vi "OpenBling.vi"(4 "OfflineMode":bool, 6 "Synchronous":bool=TRUE, 7 "Value Width":enum16{"4-bit", "8-bit"}(ring), 8 "error in (no error)":errorcluster, 9 "Chain Setup":cluster{"ChainNumber":u8, "numLeds":u8}[](array[cluster]), 10 "Reset on open?":bool, 11 "Serial Port":refnum<visa-resource-name>) -> (0 "error out":errorcluster, 3 "ControlState":T1 {"ChainMask" format="0x%02x"})   [LabVIEW 2023, in "ArduinoSerialBling.lvlib"]
uses:
  ArduinoSerialBling.lvlib
  ControlState.ctl
  ChainState.ctl
  <vilib>/Instr/_visa.llb/VISA Flush IO Buffer Mask.ctl
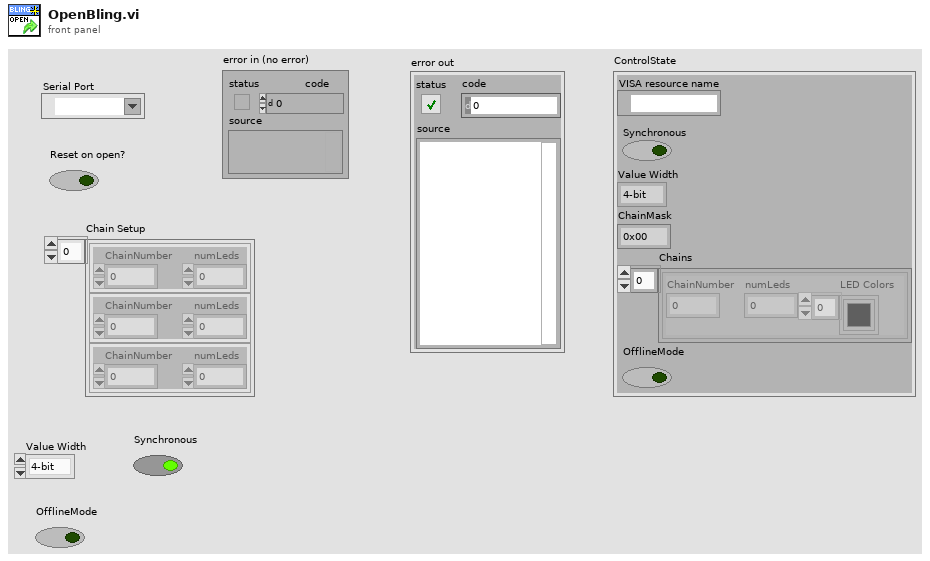
[diagram p1: front panel]
types:
  T1 = typedef "ArduinoSerialBling.lvlib/ControlState.ctl" = cluster{"VISA resource name":refnum<visa-resource-name>, "Synchronous":bool, "Value Width":enum16{"4-bit", "8-bit"}, "ChainMask":u8, "Chains":T2[], "OfflineMode":bool}
  T2 = typedef "ArduinoSerialBling.lvlib/ChainState.ctl" = cluster{"ChainNumber":u8, "numLeds":u8, "LED Colors":u32[]}
  T3 = typedef "VISA Flush IO Buffer Mask.ctl" = u16
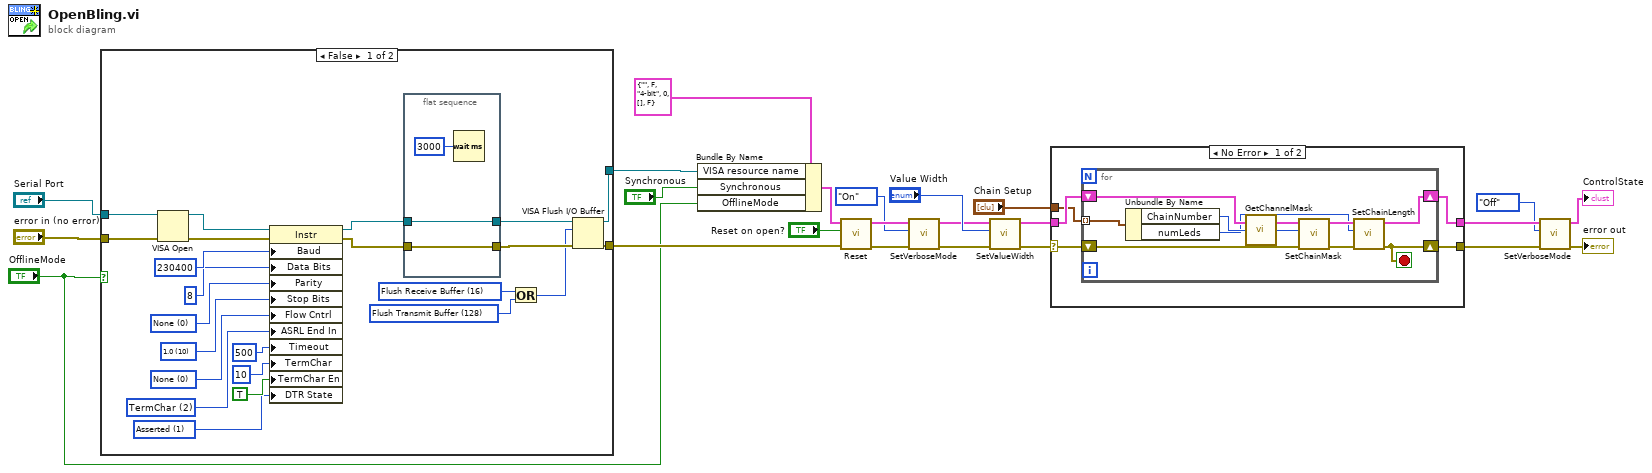
[diagram p0: block diagram]
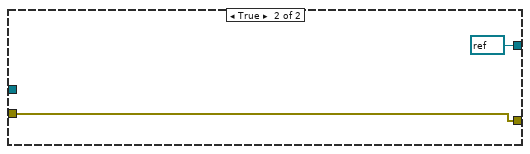
[diagram p2: hidden frame]
diagram:
  n1 = case shown="False" "OfflineMode" {
    tunnel: [w44 refnum<visa-resource-name> refnum ("Serial Port")] -> w5
    tunnel: [w43 w51] -> w4
    tunnel: "Serial Port" -> [w39 _]
    tunnel: "error in (no error)" -> [w25 w51]
    frame False {
      w26 = i16 1 items=["Unknown"=-1, "Unasserted"=0, "Asserted"=1] ("Serial Settings:Modem Line Settings:Line DTR State")
      w32 = u16 2 items=["None", "Last Bit", "TermChar"] ("Serial Settings:End Mode for Reads")
      w33 = u16 0 items=["None", "XON/XOFF", "RTS/CTS", "XON/XOFF & RTS/CTS", "DTR/DSR", "XON/XOFF & DTR/DSR"] ("Serial Settings:Flow Control")
      w34 = u16 10 items=["1.0"=10, "1.5"=15, "2.0"=20] ("Serial Settings:Stop Bits")
      w35 = u16 0 items=["None", "Odd", "Even", "Mark", "Space"] ("Serial Settings:Parity")
      w40 = T3 128 items=["Flush Receive Buffer"=16, "Write Transmit Buffer to Device"=32, "Flush Receive Buffer (No I/O)"=64, "Flush Transmit Buffer"=128] ("y")
      w42 = T3 16 items=["Flush Receive Buffer"=16, "Write Transmit Buffer to Device"=32, "Flush Receive Buffer (No I/O)"=64, "Flush Transmit Buffer"=128] ("Mask")
      n2 = VISA Open(error in (no error)=w25, VISA resource name=w39) -> (VISA resource name=w38:refnum<visa-resource-name>, error out=w24:errorcluster)  [unwired: 3 in]
      n3 = property class="Instr"(reference=w38, error in=w24, "Baud"=u32 230400 ("baud rate (9600)"), "Data Bits"=u16 8 ("Serial Settings:Data Bits"), "Parity"=w35, "Stop Bits"=w34, "Flow Cntrl"=w33, "ASRL End In"=w32, "Timeout"=u32 500 ("timeout (10sec)"), "TermChar"=u8 10 ("Message Based Settings:Termination Character"), "TermChar En"=TRUE ("Message Based Settings:Termination Character Enable"), "DTR State"=w26) -> (reference out=w28:refnum<visa-resource-name>, error out=w27:errorcluster)
      n4 = flat-sequence {
        tunnel: [w49] -> w45
        tunnel: w27 -> [w49]
        tunnel: [w48] -> w46
        tunnel: w28 -> [w48]
        frame #0 {
          n5 = Wait (ms)(milliseconds to wait=u32 3000) -> ()  [unwired: 1 out]
        }
      }
      n6 = Or(x=w42, y=w40) -> (x .or. y?=w41:T3)
      n7 = VISA Flush I/O Buffer(VISA resource name=w46, mask (16)=w41, error in (no error)=w45) -> (VISA resource name out=w44:refnum<visa-resource-name>, error out=w43:errorcluster)
    }
    frame True {
    }
  }
  n8 = Bundle By Name(cluster=T1 {"VISA resource name"="", "Synchronous"=FALSE, "Value Width"=enum."4-bit", "ChainMask"=0, "Chains"=[], "OfflineMode"=FALSE} ("ControlState"), "VISA resource name"=w5, "Synchronous"="Synchronous", "OfflineMode"="OfflineMode") -> (w21:T1)
  n9 = call "Reset.vi"("error in (no error)"=w4, "Reset"="Reset on open?", "ControlState in"=w21) -> ("error out"=w15:errorcluster, "ControlState out"=w16:T1)  [unwired: 7 in]
  n10 = call "SetVerboseMode.vi"("error in (no error)"=w15, "Verbosity"=enum16{"Off", "On"}."On", "ControlState in"=w16) -> ("error out"=w14:errorcluster, "ControlState out"=w12:T1)  [unwired: 7 in]
  n11 = call "SetValueWidth.vi"("error in (no error)"=w14, "Value Width"="Value Width", "ControlState in"=w12) -> ("error out"=w19:errorcluster, "ControlState out"=w18:T1)  [unwired: 7 in]
  n12 = case shown="No Error" w19 {
    selector: w19 -> [w56 w67]
    tunnel: w18 -> [w55 w68]
    tunnel: "Chain Setup" -> [w54 _]
    tunnel: [w53 w68] -> w11
    tunnel: [w52 w67] -> w10
    frame No Error {
      n13 = for {
        tunnel: w54 -> [w64] mode=indexing
        shift-right: [w57] -> w53
        shift-left: w55 -> [w66]
        shift-right: [w58] -> w52
        shift-left: w56 -> [w62]
        stop <- w58 stop-if-true
        n14 = Unbundle By Name(w64) -> ("ChainNumber"=w63:u8, "numLeds"=w60:u8)
        n15 = call "GetChannelMask.vi"("ChainNumber"=w63) -> ("ChainMask"=w65:u8)
        n16 = call "SetChainMask.vi"("error in (no error)"=w62, "ChainMask"=w65, "ControlState in"=w66) -> ("error out"=w59:errorcluster, "ControlState out"=w61:T1)  [unwired: 7 in]
        n17 = call "SetChainLength.vi"("error in (no error)"=w59, "Chain Length"=w60, "ControlState in"=w61) -> ("error out"=w58:errorcluster, "ControlState out"=w57:T1)  [unwired: 7 in]
      }
    }
    frame Error {
    }
  }
  n18 = call "SetVerboseMode.vi"("error in (no error)"=w10, "Verbosity"=enum16{"Off", "On"}."Off", "ControlState in"=w11) -> ("error out"=→"error out":errorcluster, "ControlState out"=→"ControlState":T1)  [unwired: 7 in]
